vi "Get UIConfiguration_lvclass.vi"(8 "error in (no error)":errorcluster, 11 "ScriptDialog in":refnum<class "ScriptDialog.lvclass">) -> (0 "error out":errorcluster, 2 "UIConfiguration.lvclass":refnum<class "UIConfiguration.lvclass">, 3 "ScriptDialog out":refnum<class "ScriptDialog.lvclass">)   [LabVIEW 2015, in "ScriptDialog.lvclass"]
uses:
  ScriptDialog.lvclass
  System/UIConfiguration/UIConfiguration.lvclass
  ScriptDialog.lvclass/ScriptDialog.ctl
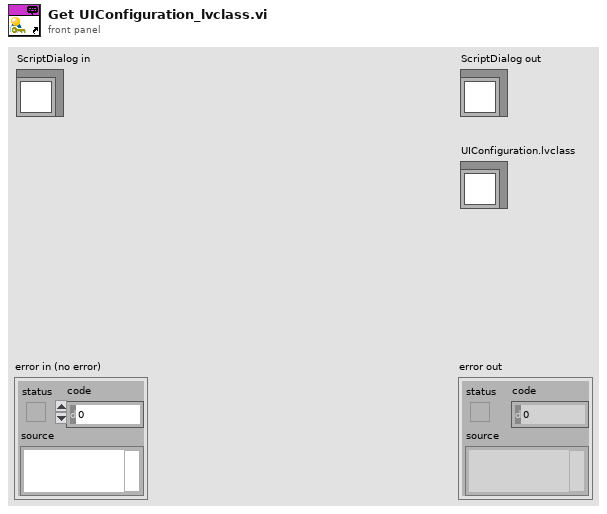
[diagram p1: front panel]
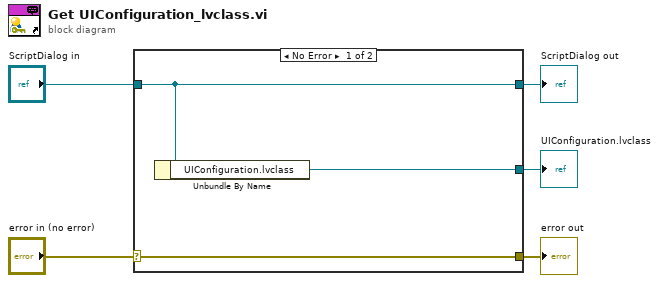
[diagram p0: block diagram]
diagram:
  n1 = case shown="No Error" "error in (no error)" {
    selector: "error in (no error)" -> [w8 w9]
    tunnel: [w8 w9] -> w4
    tunnel: [w7 w10] -> w2
    tunnel: "ScriptDialog in" -> [w7 w10]
    tunnel: [w6 _] -> w1
    frame No Error {
      n2 = Unbundle By Name(w7) -> ("UIConfiguration.lvclass"=w6:refnum<class "UIConfiguration.lvclass">)
    }
    frame Error {
    }
  }
  "error out" <- w4
  "ScriptDialog out" <- w2
  "UIConfiguration.lvclass" <- w1
